vi "模拟量采集配置.vi"() -> (3 "DeviceID":i32)   [LabVIEW 2013]
uses:
  C:/ART/PCI8622/Driver/INF/XP/i386/PCI862232.dll
panel:
  in  "AD模式选择":i32(ring) items=["连续采样", "分组采样"]
  in  "程控增益":i32(ring) items=["1倍增益", "2倍增益", "5倍增益", "10倍增益"]
  in  "触发方式":i32(ring) items=["内触发", "后触发"]
  in  "触发类型":i32(ring) items=["边沿触发", "脉冲触发"]
  in  "分组循环次数":i32=1 min=0 max=255
  in  "触发方向":i32(ring) items=["负向触发", "正向触发", "正负向触发"]
  in  "时钟输出":i32(ring) items=["禁止", "允许"]
  in  "时钟源选择":i32(ring) items=["内时钟", "外时钟"]
  in  "采样频率(Hz)":i32=200000 min=0 max=250000
  in  "分组间隔(uS)":i32=100 min=0 max=419430
  in  "触发灵敏窗(25nS)":i32=100 min=1 max=65535
  in  "超时时间(秒)":i32 min=0 max=3600
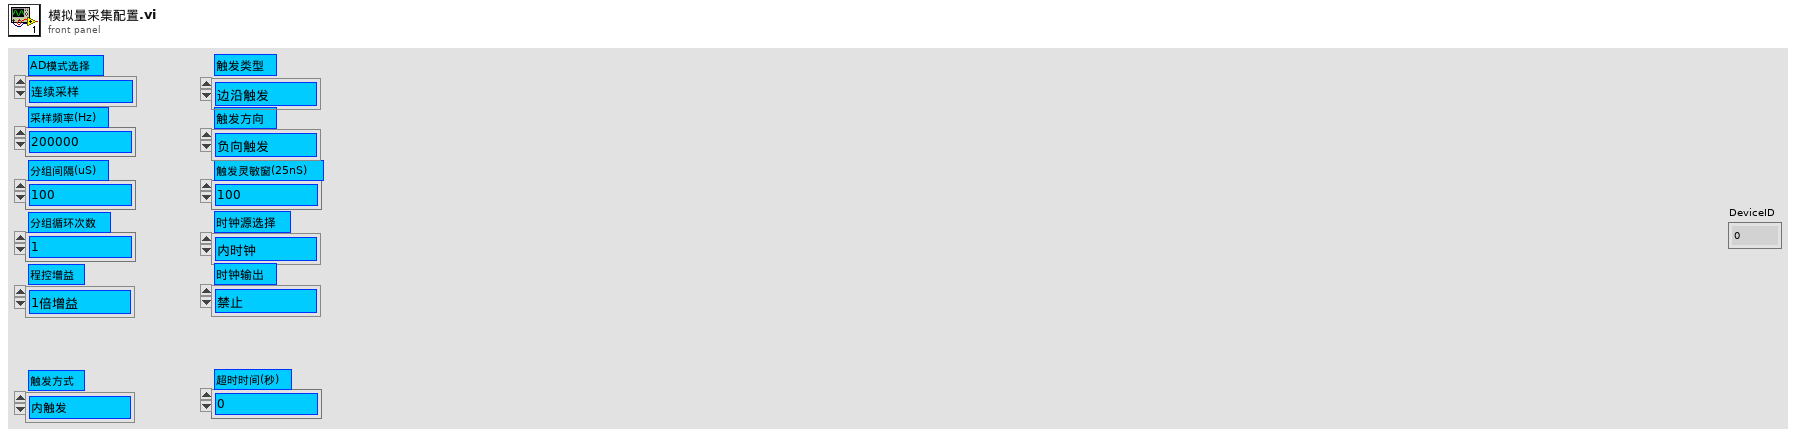
[diagram p1: front panel]
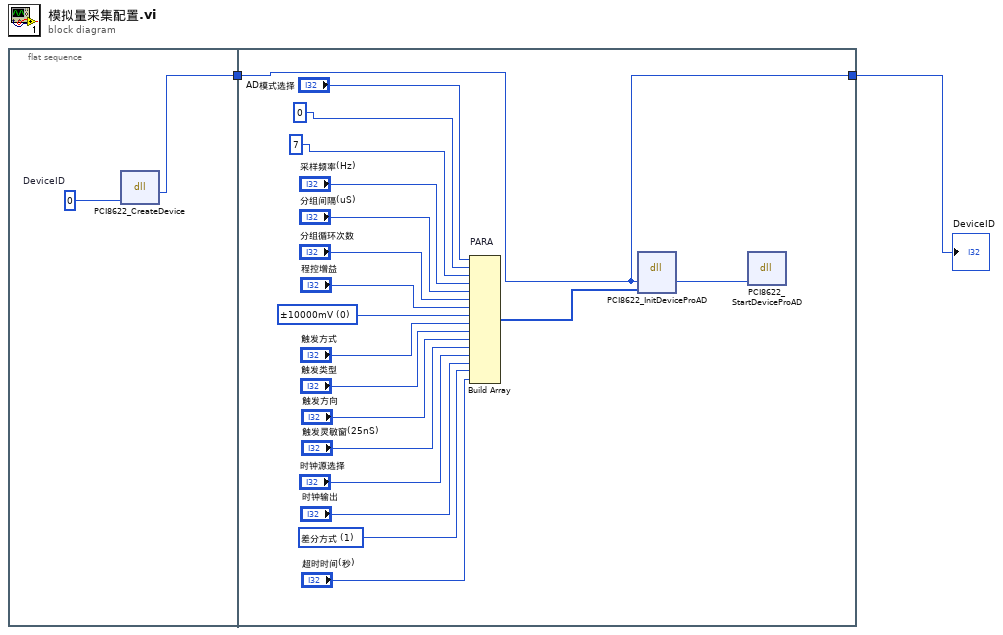
[diagram p0: block diagram]
diagram:
  n1 = flat-sequence {
    tunnel: [w4] -> w2
    tunnel: w2 -> [w6]
    tunnel: [w6] -> w1
    frame #0 {
      w3 = 0  # DeviceID
      n2 = dll-call lib="C:/ART/PCI8622/Driver/INF/XP/i386/PCI862232.dll" fn="PCI8622_CreateDevice" label="CreateDevice"("DeviceID"=w3) -> ("返回类型"=w4:i32)  [unwired: 4 in, 2 out]
    }
    frame #1 {
      w5 = 1 items=["单端方式", "差分方式"] ("接地方式")
      w7 = 0 items=["±10000mV", "±5000mV", "±2500mV", "0～10000mV", "0～5000mV"] ("量程范围")
      n3 = Build Array "PARA"("AD模式选择", 0 ("首通道"), 7 ("末通道"), "采样频率(Hz)", "分组间隔(uS)", "分组循环次数", "程控增益", w7, "触发方式", "触发类型", "触发方向", "触发灵敏窗(25nS)", "时钟源选择", "时钟输出", w5, "超时时间(秒)") -> (w16:i32[])
      n4 = dll-call lib="C:/ART/PCI8622/Driver/INF/XP/i386/PCI862232.dll" fn="PCI8622_InitDeviceProAD" label="InitDeviceProAD"("hDevice"=w6, "pADPara"=w16) -> ("hDevice"=w10:i32)  [unwired: 5 in, 2 out]
      n5 = dll-call lib="C:/ART/PCI8622/Driver/INF/XP/i386/PCI862232.dll" fn="PCI8622_StartDeviceProAD" label="StartDeviceProAD"("hDevice"=w10) -> ()  [unwired: 5 in, 2 out]
    }
  }
  "DeviceID" <- w1
